vi "Start Sync.vi"(8 "error in":errorcluster, 11 "gRPC Server in":refnum<class "NW and PSD_server.lvclass">) -> (0 "error out":errorcluster, 3 "gRPC Server out":refnum<class "NW and PSD_server.lvclass">)   [LabVIEW 2019, in "NW and PSD_server.lvlib" / "NW and PSD_server.lvclass"]
uses:
  NW and PSD_server.lvclass
  RPC Messages/example_SignalParameters/example_SignalParameters_Data.ctl
  RPC Messages/example_SamplingInfo/example_SamplingInfo_Data.ctl
  RPC Messages/example_NoiseParameters/example_NoiseParameters_Data.ctl
  RPC Messages/example_AnalyzedResults/example_AnalyzedResults_Data.ctl
  NW and PSD_server.lvclass/NW and PSD_server.ctl
  RPC Messages/example_noData/example_noData_Data.ctl
  <vilib>/measure/NI_MABase.lvlib
  <vilib>/measure/NI_MAPro.lvlib
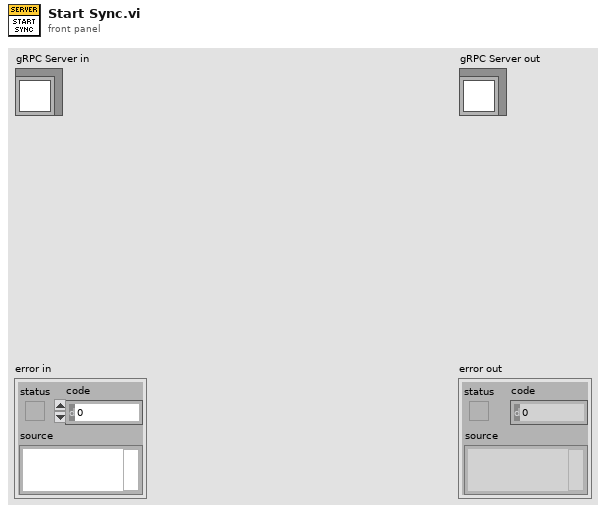
[diagram p1: front panel]
types:
  T1 = typedef "NW and PSD_server.lvlib/NW and PSD_server.lvclass/example_noData_Data.ctl" = cluster{"response":string}
  T2 = cluster{"lower cutoff freq":dbl, "higher cutoff freq":dbl, "order":i32}
  T3 = typedef "NW and PSD_server.lvlib/NW and PSD_server.lvclass/example_AnalyzedResults_Data.ctl" = cluster{"sinad":sgl, "THD_plus_noise":sgl}
  T4 = typedef "NW and PSD_server.lvlib/NW and PSD_server.lvclass/example_NoiseParameters_Data.ctl" = cluster{"sampling_info":T5, "noiseamplitude":sgl, "noisetype":i32}
  T5 = typedef "NW and PSD_server.lvlib/NW and PSD_server.lvclass/example_SamplingInfo_Data.ctl" = cluster{"number_of_samples":i32, "sample_rate":sgl}
  T6 = typedef "NW and PSD_server.lvlib/NW and PSD_server.lvclass/example_SignalParameters_Data.ctl" = cluster{"sampling_info":T5, "frequency":sgl, "amplitude":sgl}
  T7 = typedef "NW and PSD_server.lvlib/NW and PSD_server.lvclass/Server gRPC UEs.ctl" = cluster{"example_SignalGeneratorService_ApplySignalParameters gRPC UE":refnum<user-event>, "example_SignalGeneratorService_ApplyNoiseParameters gRPC UE":refnum<user-event>, "example_SignalGeneratorService_GenerateSignal gRPC UE":refnum<user-event>, "example_SignalGeneratorService_GetAnalyzedParameters gRPC UE":refnum<user-event>}
  T8 = cluster{"Signal Parameter":T6, "Noise Parameter":T4, "Measured Parameter":T3}
  T9 = typedef "gprc-lvsupport-release.lvlib/grpcId.ctl" = u64
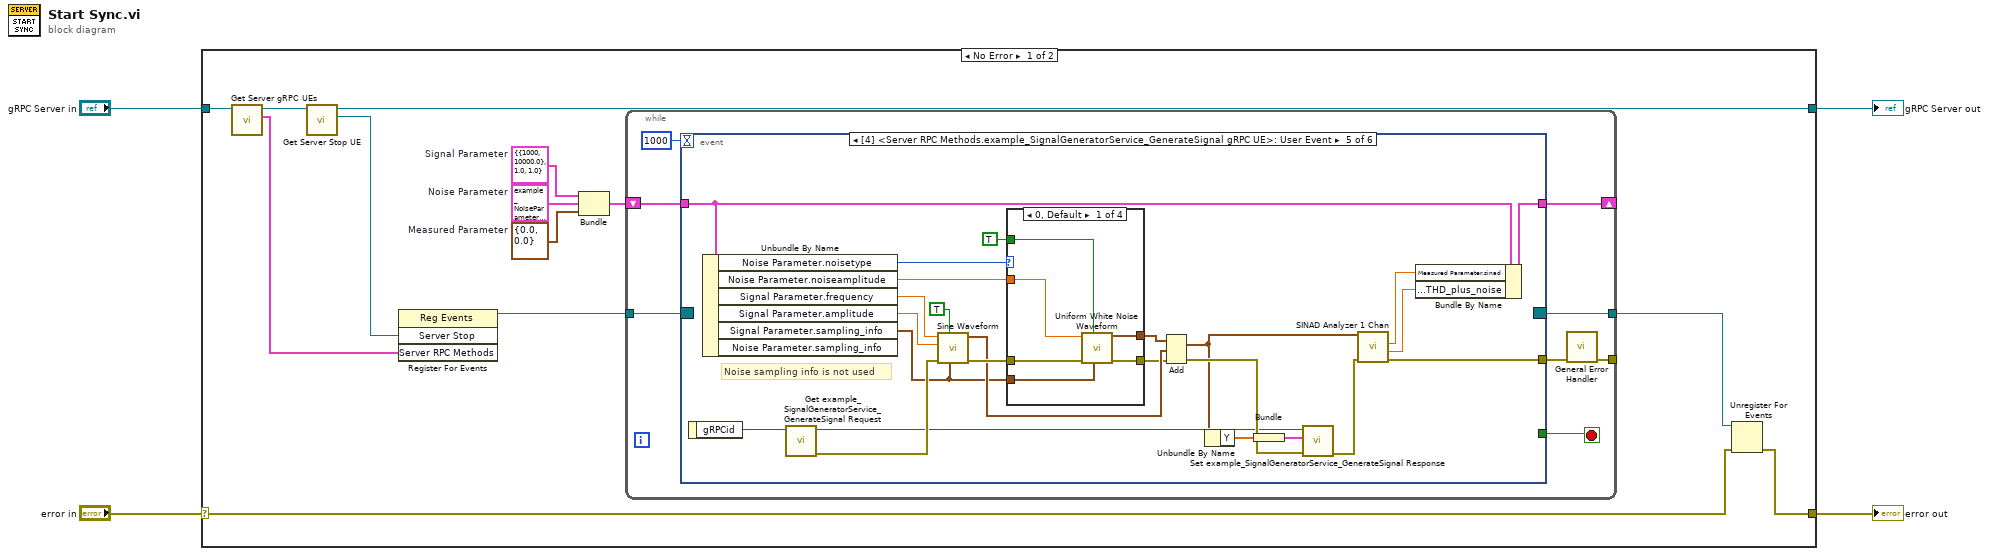
[diagram p0: block diagram]
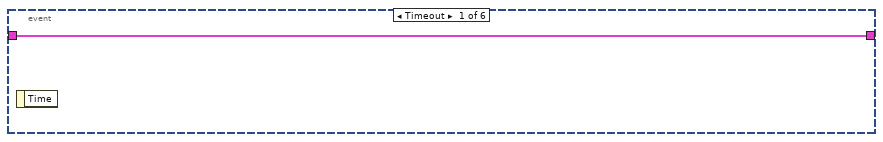
[diagram p2: hidden frame]
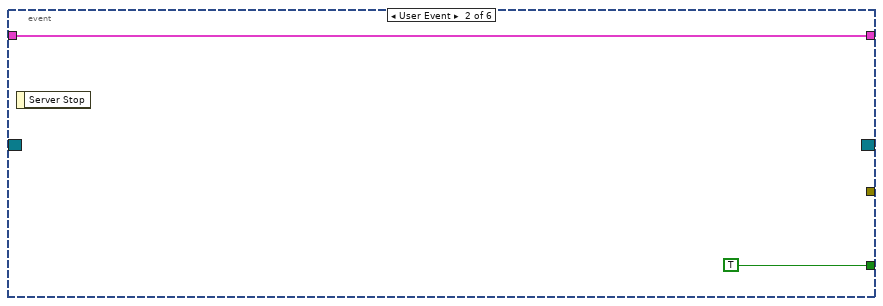
[diagram p3: hidden frame]
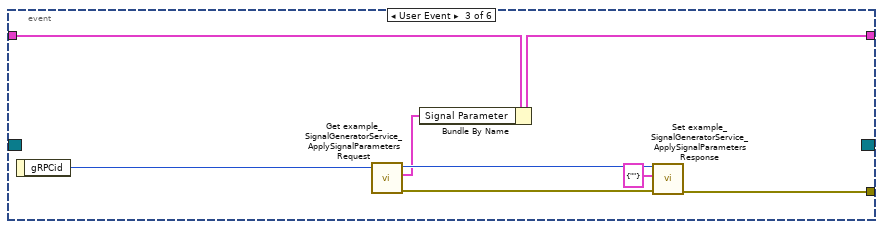
[diagram p4: hidden frame]
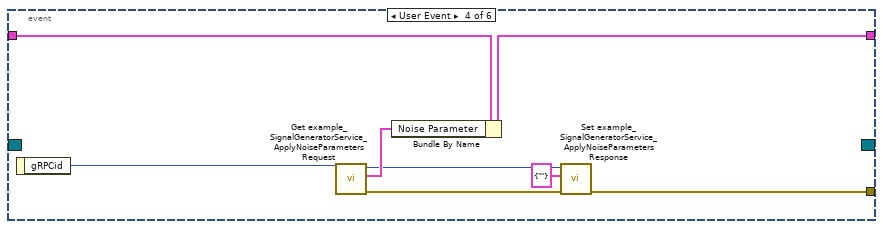
[diagram p5: hidden frame]
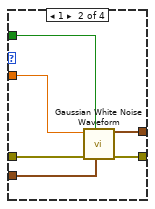
[diagram p6: hidden frame]
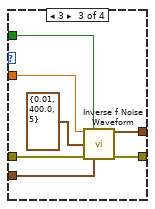
[diagram p7: hidden frame]
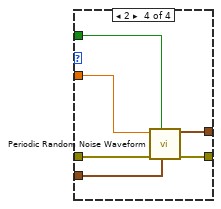
[diagram p8: hidden frame]
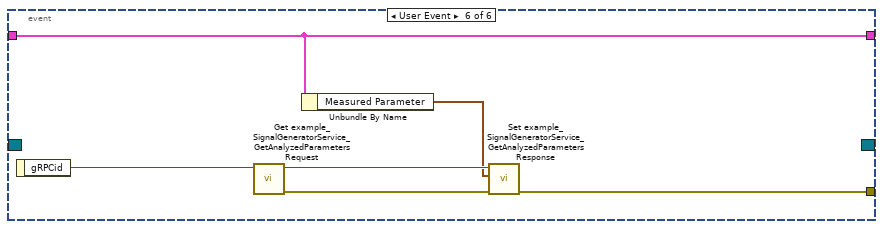
[diagram p9: hidden frame]
diagram:
  n1 = case shown="No Error" "error in" {
    selector: "error in" -> [w10 w101]
    tunnel: [w9 w101] -> w3
    tunnel: [w13 w100] -> w1
    tunnel: "gRPC Server in" -> [w17 w100]
    frame No Error {
      w5 = T3 {"sinad"=0.0, "THD_plus_noise"=0.0}  # Measured Parameter
      w6 = T4 {"sampling_info"={"number_of_samples"=1000, "sample_rate"=10000.0}, "noiseamplitude"=0.1, "noisetype"=3}  # Noise Parameter
      w8 = T6 {"sampling_info"={"number_of_samples"=1000, "sample_rate"=10000.0}, "frequency"=1.0, "amplitude"=1.0}  # Signal Parameter
      n2 = call "Get Server gRPC UEs.vi"("OOP Server in"=w17) -> ("Server RPC Methods"=w14:T7, "OOP Server out"=w16:refnum<class "NW and PSD_server.lvclass">)  [unwired: 9 in]
      n3 = call "Get Server Stop UE.vi"("OOP Server in"=w16) -> ("Server Stop"=w15:refnum<user-event>, "OOP Server out"=w13:refnum<class "NW and PSD_server.lvclass">)  [unwired: 9 in]
      n4 = register-events(w15, w14) -> (reference out=w12:refnum<event-registration>)  [unwired: 2 in, 1 out]
      n5 = Bundle("Signal Parameter"=w8, "Noise Parameter"=w6, "Measured Parameter"=w5) -> (w7:T8)  [unwired: 1 in]
      n6 = while {
        tunnel: w12 -> [w25]
        tunnel: [w23] -> w11
        tunnel: [w20] -> _
        shift-right: [w18] -> _
        shift-left: w7 -> [w19]
        stop <- w24 stop-if-true
        n7 = event "RPC Methods Event Structure" shown="[4] <Server RPC Methods.example_SignalGeneratorService_GenerateSignal gRPC UE>: User Event" {
          selector: w25 -> [_ _ _ _ _ _]
          dyn-events: [_ _ _ _ _ _] -> w23
          timeout: 1000 -> [_ _ _ _ _ _]
          tunnel: [_ TRUE _ _ _ _] -> w24
          tunnel: [_ _ w33 w38 w51 w96] -> w21
          tunnel: w19 -> [w26 w27 w31 w41 w49 w95]
          tunnel: [w26 w27 w29 w42 w48 w95] -> w18
          event Timeout {
            n8 = event-data() -> ()  [unwired: 1 in, 1 out]
          }
          event User Event {
            n9 = event-data() -> ()  [unwired: 1 in, 1 out]
          }
          event User Event {
            n10 = event-data() -> ("gRPCid"=w36:T9)  [unwired: 1 in]
            n11 = call "Get example_SignalGeneratorService_ApplySignalParameters Request.vi"("gRPCid in"=w36) -> ("error out"=w34:errorcluster, "Message Data"=w30:T6, "gRPCid out"=w35:T9)  [unwired: 8 in]
            n12 = Bundle By Name(cluster=w31, "Signal Parameter"=w30) -> (w29:T8)
            n13 = call "Set example_SignalGeneratorService_ApplySignalParameters Response.vi"("error in (no error)"=w34, "Message Data"=T1 {"response"=""}, "gRPCid in"=w35) -> ("error out"=w33:errorcluster)  [unwired: 8 in]
          }
          event User Event {
            n14 = event-data() -> ("gRPCid"=w44:T9)  [unwired: 1 in]
            n15 = call "Get example_SignalGeneratorService_ApplyNoiseParameters Request.vi"("gRPCid in"=w44) -> ("error out"=w40:errorcluster, "Message Data"=w43:T4, "gRPCid out"=w39:T9)  [unwired: 8 in]
            n16 = Bundle By Name(cluster=w41, "Noise Parameter"=w43) -> (w42:T8)
            n17 = call "Set example_SignalGeneratorService_ApplyNoiseParameters Response.vi"("error in (no error)"=w40, "Message Data"=T1 {"response"=""}, "gRPCid in"=w39) -> ("error out"=w38:errorcluster)  [unwired: 8 in]
          }
          event User Event {
            # "Noise sampling info is not used"
            n18 = event-data() -> ("gRPCid"=w68:T9)  [unwired: 1 in]
            n19 = Unbundle By Name(w49) -> ("Noise Parameter.noisetype"=w62:i32, "Noise Parameter.noiseamplitude"=w63:sgl, "Signal Parameter.frequency"=w65:sgl, "Signal Parameter.amplitude"=w64:sgl, "Signal Parameter.sampling_info"=w45:T5)  [unwired: 1 out]
            n20 = call "Get example_SignalGeneratorService_GenerateSignal Request.vi"("gRPCid in"=w68) -> ("error out"=w56:errorcluster, "gRPCid out"=w55:T9)  [unwired: 8 in, 1 out]
            n21 = call <vilib>:"Sine Waveform.vi"("sampling info"=w45, "reset signal"=TRUE, "error in (no error)"=w56, "amplitude"=w64, "frequency"=w65) -> ("error out"=w67:errorcluster, "signal out"=w59:waveform(dbl))  [unwired: 5 in]
            n22 = case shown="0, Default" w62 {
              tunnel: w67 -> [w74 w80 w87 w93]
              tunnel: w45 -> [w73 w79 w86 w92]
              tunnel: TRUE ("reset signal") -> [w69 w78 w85 w88]
              tunnel: w63 -> [w72 w77 w84 w91]
              tunnel: [w71 w76 w83 w90] -> w60
              tunnel: [w70 w75 w82 w89] -> w58
              frame 0, Default {
                n23 = call <vilib>:"Uniform White Noise Waveform.vi"("sampling info"=w73, "reset signal"=w69, "error in (no error)"=w74, "amplitude"=w72) -> ("error out"=w70:errorcluster, "signal out"=w71:waveform(dbl))  [unwired: 6 in]
              }
              frame 1 {
                n24 = call <vilib>:"Gaussian White Noise Waveform.vi"("sampling info"=w79, "reset signal"=w78, "error in (no error)"=w80, "standard deviation"=w77) -> ("error out"=w75:errorcluster, "signal out"=w76:waveform(dbl))  [unwired: 6 in]
              }
              frame 3 {
                n25 = call <vilib>:"Inverse f Noise Waveform.vi"("noise density"=w84, "reset signal (F)"=w85, "filter specifications"=T2 {"lower cutoff freq"=0.01, "higher cutoff freq"=400.0, "order"=5}, "error in (no error)"=w87, "sampling info"=w86) -> ("signal out"=w83:waveform(dbl), "error out"=w82:errorcluster)  [unwired: 6 in, 3 out]
              }
              frame 2 {
                n26 = call <vilib>:"Periodic Random Noise Waveform.vi"("sampling info"=w92, "reset signal"=w88, "error in (no error)"=w93, "spectral amplitude"=w91) -> ("error out"=w89:errorcluster, "signal out"=w90:waveform(dbl))  [unwired: 6 in]
              }
            }
            n27 = Add(1:w59, 2:w60, 4:w58) -> (0:w50:waveform(dbl), 3:w57:errorcluster)
            n28 = Unbundle By Name(w50) -> ("Y"=w54:dbl[])
            n29 = Bundle("Y"=w54) -> (w53:cluster{"Y":dbl[]})  [unwired: 1 in]
            n30 = call "Set example_SignalGeneratorService_GenerateSignal Response.vi"("error in (no error)"=w57, "Message Data"=w53, "gRPCid in"=w55) -> ("error out"=w52:errorcluster)  [unwired: 8 in]
            n31 = call <vilib>:"SINAD Analyzer 1 Chan.vi"("error in (no error)"=w52, "signal in"=w50) -> ("error out"=w51:errorcluster, "THD Plus Noise"=w46:dbl, "SINAD (dB)"=w47:dbl)  [unwired: 4 in, 3 out]
            n32 = Bundle By Name(cluster=w49, "Measured Parameter.sinad"=w47, "Measured Parameter.THD_plus_noise"=w46) -> (w48:T8)
          }
          event User Event {
            n33 = event-data() -> ("gRPCid"=w99:T9)  [unwired: 1 in]
            n34 = call "Get example_SignalGeneratorService_GetAnalyzedParameters Request.vi"("gRPCid in"=w99) -> ("error out"=w97:errorcluster, "gRPCid out"=w98:T9)  [unwired: 8 in, 1 out]
            n35 = Unbundle By Name(w95) -> ("Measured Parameter"=w94:T3)
            n36 = call "Set example_SignalGeneratorService_GetAnalyzedParameters Response.vi"("error in (no error)"=w97, "Message Data"=w94, "gRPCid in"=w98) -> ("error out"=w96:errorcluster)  [unwired: 8 in]
          }
        }
        n37 = call <vilib>:"General Error Handler.vi"("error in (no error)"=w21) -> ("error out"=w20:errorcluster)  [unwired: 10 in, 4 out]
      }
      n38 = Unregister For Events(event registration refnum=w11, error in=w10) -> (error out=w9:errorcluster)
    }
    frame Error {
    }
  }
  "error out" <- w3
  "gRPC Server out" <- w1
